vi "visitDot.vi"(8 "error in (no error)":errorcluster, 10 "Dot":refnum<class "Dot.lvclass">, 11 "XMLExportVisitor in":refnum<class "XMLExportVisitor.lvclass">) -> (0 "error out":errorcluster, 2 "xml String":string, 3 "XMLExportVisitor out":refnum<class "XMLExportVisitor.lvclass">)   [LabVIEW 2017, in "XMLExportVisitor.lvclass"]
uses:
  XMLExportVisitor.lvclass
  Dot Class/Dot.lvclass
  Dot Class/Dot.lvclass/Dot.ctl
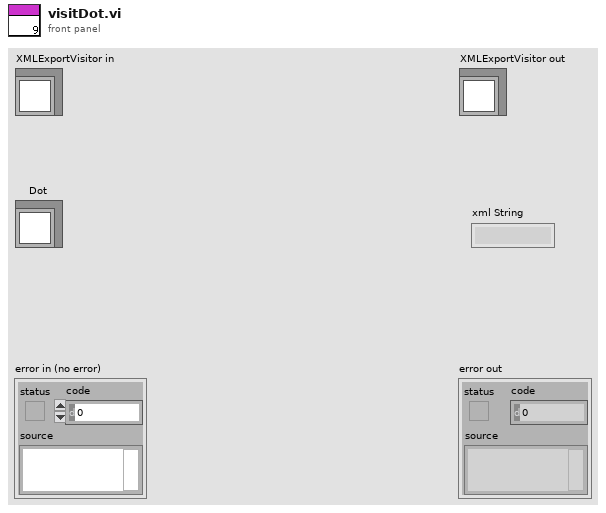
[diagram p1: front panel]
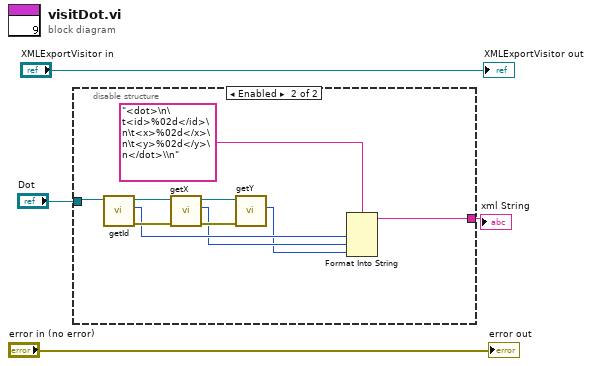
[diagram p0: block diagram]
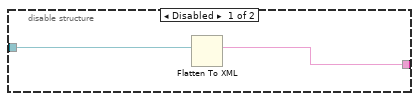
[diagram p2: hidden frame]
diagram:
  n1 = disable-structure shown="Enabled" {
    disable-tunnel: [w6 w7] -> w2
    disable-tunnel: "Dot" -> [w5 w16]
    frame Disabled {
      n2 = Flatten To XML(anything=w5) -> (xml string=w6:string)
    }
    frame Enabled {
      n3 = call "getId.vi"("Dot in"=w16) -> ("error out"=w14:errorcluster, "id"=w10:i32, "Dot out"=w15:refnum<class "Dot.lvclass">)  [unwired: 8 in]
      n4 = call "getX.vi"("error in (no error)"=w14, "Dot in"=w15) -> ("error out"=w12:errorcluster, "x"=w9:i32, "Dot out"=w13:refnum<class "Dot.lvclass">)  [unwired: 7 in]
      n5 = call "getY.vi"("error in (no error)"=w12, "Dot in"=w13) -> ("y"=w8:i32)  [unwired: 7 in, 2 out]
      n6 = Format Into String(format string="<dot>\n\t<id>%02d</id>\n\t<x>%02d</x>\n\t<y>%02d</y>\n</dot>\\n", w10, w9, w8) -> (resulting string=w7:string)  [unwired: 2 in, 1 out]
    }
  }
  "xml String" <- w2
  "error out" <- "error in (no error)"
  "XMLExportVisitor out" <- "XMLExportVisitor in"
